vi "gate increment.vi"(10 "Increment":dbl, 11 "Gate Voltage":dbl) -> ()   [LabVIEW 2010]
panel:
  in  "Voltage Safety Limit":dbl
  # "Gate Increment"
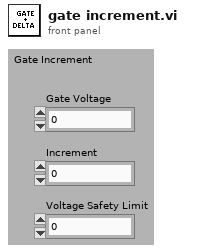
[diagram p1: front panel]
types:
  T1 = enum16{"Set Voltage", "Read Voltage", "Read Setpoint", "Read Current", "Output On", "Output Off"}
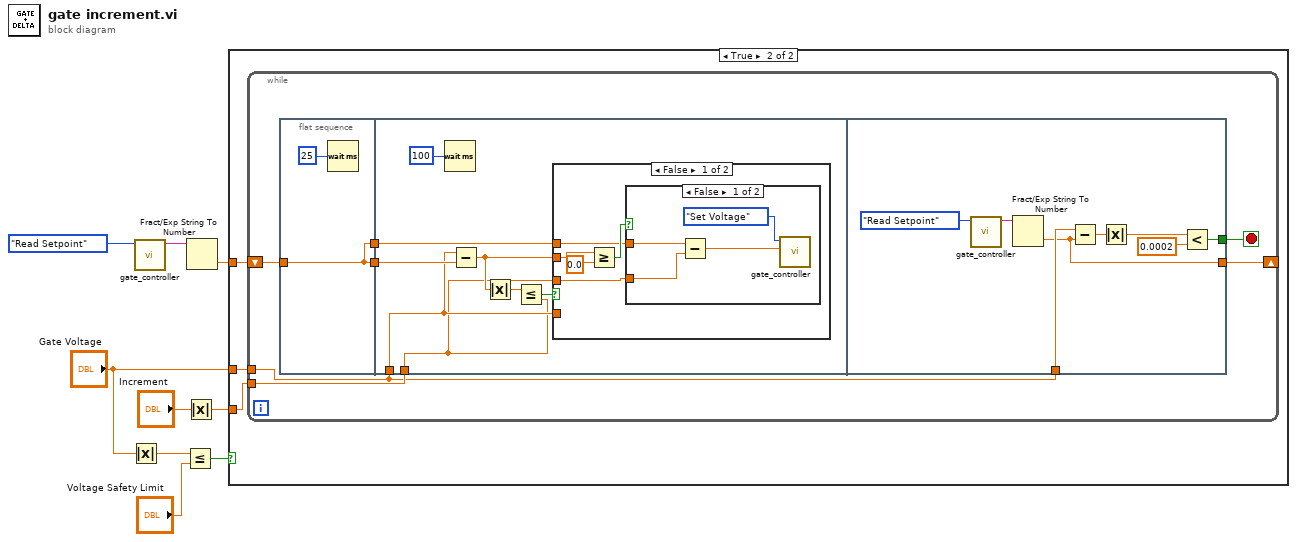
[diagram p0: block diagram]
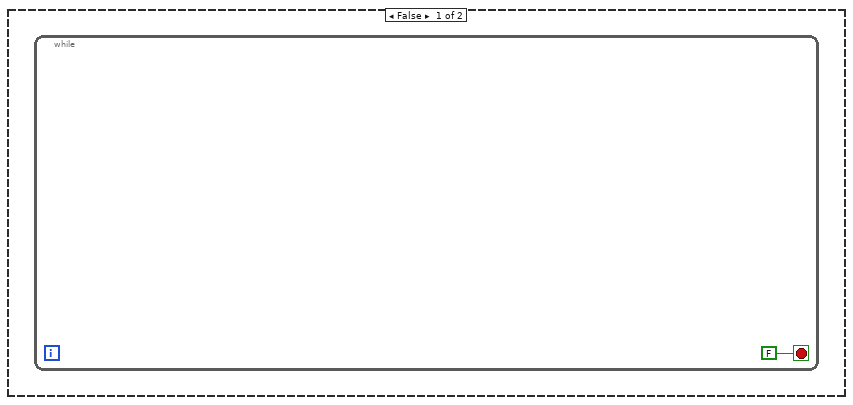
[diagram p2: hidden frame]
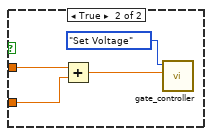
[diagram p3: hidden frame]
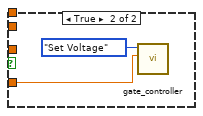
[diagram p4: hidden frame]
diagram:
  n1 = Absolute Value(x="Gate Voltage") -> (abs(x)=w5:dbl)
  n2 = call "gate_controller.vi"("Command"=T1."Read Setpoint") -> ("Response"=w9:string)  [unwired: 10 in]
  n3 = Less Or Equal?(x=w5, y="Voltage Safety Limit") -> (x <= y?=w4:bool)
  n4 = Absolute Value(x="Increment") -> (abs(x)=w6:dbl)
  n5 = Fract/Exp String To Number(string=w9) -> (number=w7:dbl)  [unwired: 3 in, 1 out]
  n6 = case shown="True" w4 {
    tunnel: "Gate Voltage" -> [_ w13]
    tunnel: w7 -> [_ w12]
    tunnel: w6 -> [_ w11]
    frame False {
      n7 = while {
        stop <- FALSE stop-if-true
      }
    }
    frame True {
      n8 = while {
        tunnel: w13 -> [w18]
        tunnel: w11 -> [w19]
        shift-right: [w14] -> _
        shift-left: w12 -> [w15]
        stop <- w17 stop-if-true
        n9 = flat-sequence {
          tunnel: [w21] -> w20
          tunnel: [w21] -> w16
          tunnel: w15 -> [w21]
          tunnel: w18 -> [w27]
          tunnel: w20 -> [w30]
          tunnel: w19 -> [w24]
          tunnel: w16 -> [w23]
          tunnel: w18 -> [w51]
          tunnel: [w47] -> w17
          tunnel: [w46] -> w14
          frame #0 {
            n10 = Wait (ms)(milliseconds to wait=u32 25) -> ()  [unwired: 1 out]
          }
          frame #1 {
            n11 = Wait (ms)(milliseconds to wait=u32 100) -> ()  [unwired: 1 out]
            n12 = Subtract(x=w27, y=w30) -> (x-y=w25:dbl)
            n13 = Absolute Value(x=w25) -> (abs(x)=w29:dbl)
            n14 = Less Or Equal?(x=w29, y=w24) -> (x <= y?=w28:bool)
            n15 = case shown="False" w28 {
              tunnel: w27 -> [_ w44]
              tunnel: w25 -> [w32 _]
              tunnel: w24 -> [w35 _]
              tunnel: w23 -> [w31 _]
              frame False {
                n16 = Greater Or Equal?(x=w32, y=0.0) -> (x >= y?=w34:bool)
                n17 = case shown="False" w34 {
                  tunnel: w35 -> [w37 w42]
                  tunnel: w31 -> [w36 w40]
                  frame False {
                    n18 = Subtract(x=w36, y=w37) -> (x-y=w38:dbl)
                    n19 = call "gate_controller.vi"("Numerical Argument"=w38, "Command"=T1."Set Voltage") -> ()  [unwired: 9 in, 1 out]
                  }
                  frame True {
                    n20 = Add(x=w40, y=w42) -> (x+y=w41:dbl)
                    n21 = call "gate_controller.vi"("Numerical Argument"=w41, "Command"=T1."Set Voltage") -> ()  [unwired: 9 in, 1 out]
                  }
                }
              }
              frame True {
                n22 = call "gate_controller.vi"("Numerical Argument"=w44, "Command"=T1."Set Voltage") -> ()  [unwired: 9 in, 1 out]
              }
            }
          }
          frame #2 {
            n23 = call "gate_controller.vi"("Command"=T1."Read Setpoint") -> ("Response"=w52:string)  [unwired: 10 in]
            n24 = Fract/Exp String To Number(string=w52) -> (number=w46:dbl)  [unwired: 3 in, 1 out]
            n25 = Subtract(x=w51, y=w46) -> (x-y=w50:dbl)
            n26 = Absolute Value(x=w50) -> (abs(x)=w49:dbl)
            n27 = Less?(x=w49, y=0.0002) -> (x < y?=w47:bool)
          }
        }
      }
    }
  }
